vi "QueryStatus.vi"(1 "Destination":T1={"Subsystem Id"=90, "Node Id"=1, "Component Id"=1}, 3 "Source":T1={"Subsystem Id"=3, "Node Id"=1, "Component Id"=1}) -> (0 "Encoded JAUS Message":string)   [LabVIEW 2009]
uses:
  Support Files/Address.ctl
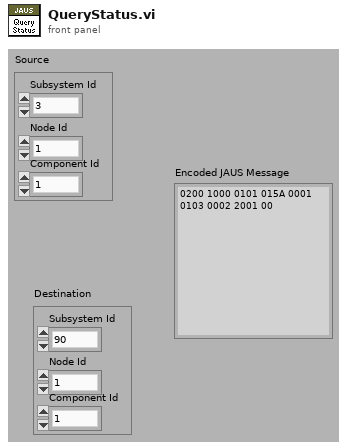
[diagram p1: front panel]
types:
  T1 = typedef "Address.ctl" = cluster{"Subsystem Id":u16, "Node Id":u8, "Component Id":u8}
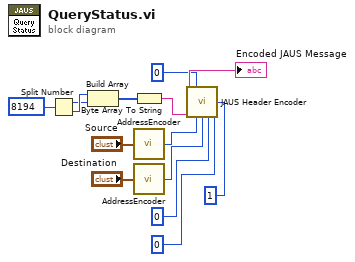
[diagram p0: block diagram]
diagram:
  n1 = Split Number(x=u16 8194 ("Message Type (0-5)")) -> (hi(x)=w3:u8, lo(x)=w4:u8)
  n2 = Build Array(w4, w3) -> (w2:u8[])
  n3 = Byte Array To String(unsigned byte array=w2) -> (string=w1:string)
  n4 = call "AddressEncoder.vi"("Address Cluster"="Source") -> ("Address"=w13:u32)
  n5 = call "AddressEncoder.vi"("Address Cluster"="Destination") -> ("Address"=w12:u32)
  n6 = call "JAUS Header Encoder.vi"("Message Type (0-5)"=u8 0, "Priority(40-41)"=u8 1, "Payload"=w1, "Source ID (80-95)"=w13, "Destination ID (48-79)"=w12, "Data Flags (46-47)"=u8 0, "Ack/Nak (44-45)"=u8 0) -> ("Encoded JAUS Message"=→"Encoded JAUS Message":string)  [unwired: 8 in]
